vi "SetNodes.vi"(0 "reference":refnum<class "StateTransitionEdge.lvclass">, 1 "Start":refnum<class "AbstractNode.lvclass">, 2 "End":refnum<class "AbstractNode.lvclass">, 5 "error in (no error)":errorcluster) -> (14 "reference out":refnum<class "StateTransitionEdge.lvclass">, 19 "error out":errorcluster)   [LabVIEW 2012, in "StateTransitionEdge.lvclass"]
doc: "SetNodes"
uses:
  <resource>/Framework/Providers/Open_GDS/UML/StateTransitionEdge_class/StateTransitionEdge.lvclass
  <resource>/Framework/Providers/Open_GDS/UML/AbstractNode_class/AbstractNode.lvclass
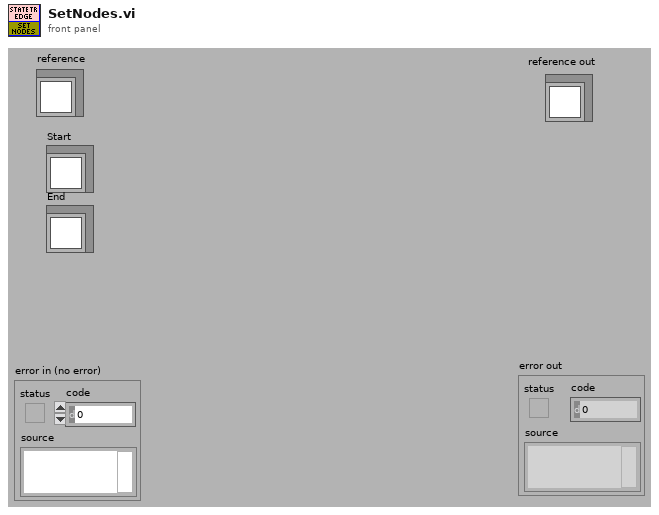
[diagram p1: front panel]
types:
  T1 = typedef "StateTransitionEdge.lvclass/ObjectAttributes.ctl" = cluster{"Base class":T2, "angle":dbl}
  T2 = typedef "ClassRelationshipEdge.lvclass/ObjectAttributes.ctl" = cluster{"Base class":T3, "bentStyleRef":refnum<class "BentStyle.lvclass">, "startConnectionOffset":cluster{"x":i32, "y":i32}, "endConnectionOffset":cluster{"x":i32, "y":i32}, "MidLineOffset":cluster{"x":i32, "y":i32}, "DepClass":T7}
  T3 = typedef "SegmentedLineEdge.lvclass/ObjectAttributes.ctl" = cluster{"Base class":T4, "lineStyle":refnum<class "LineStyle.lvclass">, "startArrowHead":refnum<class "ArrowHead.lvclass">, "endArrowHead":refnum<class "ArrowHead.lvclass">, "startLabel":string, "midLabel":string, "endLabel":string, "MidLabelOffset":T6, "SplitWire":bool}
  T4 = typedef "GeneralPathEdge.lvclass/ObjectAttributes.ctl" = cluster{"Base class":T5}
  T5 = typedef "AbstractEdge.lvclass/ObjectAttributes.ctl" = cluster{"start":refnum<class "AbstractNode.lvclass">, "end":refnum<class "AbstractNode.lvclass">}
  T6 = typedef "Point Point2D.ctl" = cluster{"x":dbl, "y":dbl}
  T7 = typedef "ReversedEngineering_ViDependencyDetailsType.ctl" = cluster{"ThisVIs/Ctls":path[], "Dependent_VIs/Ctls":path[]}
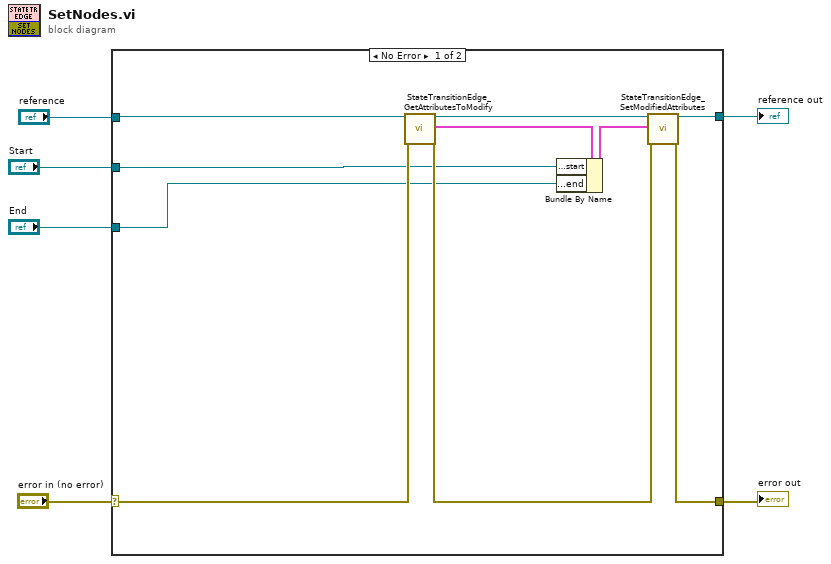
[diagram p0: block diagram]
diagram:
  n1 = case shown="No Error" "error in (no error)" {
    selector: "error in (no error)" -> [w16 w17]
    tunnel: "reference" -> [w15 w18]
    tunnel: [w10 w17] -> w4
    tunnel: [w9 w18] -> w3
    tunnel: "Start" -> [w8 _]
    tunnel: "End" -> [w7 _]
    frame No Error {
      n2 = call <resource>:"StateTransitionEdge_GetAttributesToModify.vi"("reference in"=w15, "error in (no error)"=w16) -> ("reference out"=w13:refnum<class "StateTransitionEdge.lvclass">, "Attributes"=w12:T1, "error out"=w14:errorcluster)  [unwired: 1 in, 14 out]
      n3 = Bundle By Name(cluster=w12, "Base class.Base class.Base class.Base class.start"=w8, "Base class.Base class.Base class.Base class.end"=w7) -> (w11:T1)
      n4 = call <resource>:"StateTransitionEdge_SetModifiedAttributes.vi"("reference in"=w13, "Attributes"=w11, "error in (no error)"=w14) -> ("reference out"=w9:refnum<class "StateTransitionEdge.lvclass">, "error out"=w10:errorcluster)  [unwired: 3 in, 12 out]
    }
    frame Error {
    }
  }
  "reference out" <- w3
  "error out" <- w4
